vi "Graph Utilities Tree.vi"() -> ()   [LabVIEW 2019]
uses:
  graph_utilities.lvclass/graph_utilities.ctl
  <vilib>/Analysis/baseanly.llb/A x B.vi
  <vilib>/Analysis/baseanly.llb/A x Vector.vi
  subVIs/Step Average.vi
  <vilib>/Utility/error.llb/Error Cluster From Error Code.vi
  <vilib>/PRIrvin/XY Utilities/XY to 2D.vi
  graph_utilities.lvclass
panel:
  out "Intensity Graph":dbl[][](graph)
  out "XY Graph":cluster{dbl[], dbl[]}[](graph)
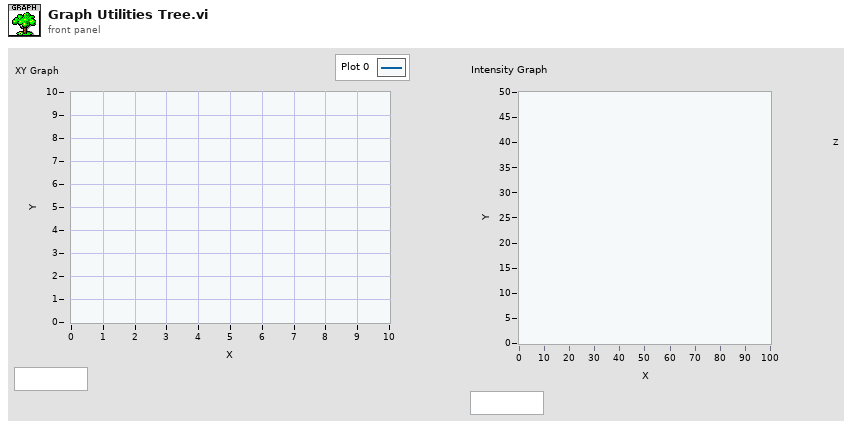
[diagram p1: front panel]
types:
  T1 = typedef "LVPointDoubleTypeDef.ctl" = cluster{"X":dbl, "Y":dbl}
  T2 = typedef "graph_utilities.lvclass/Scale Mapping --enum.ctl" = u16
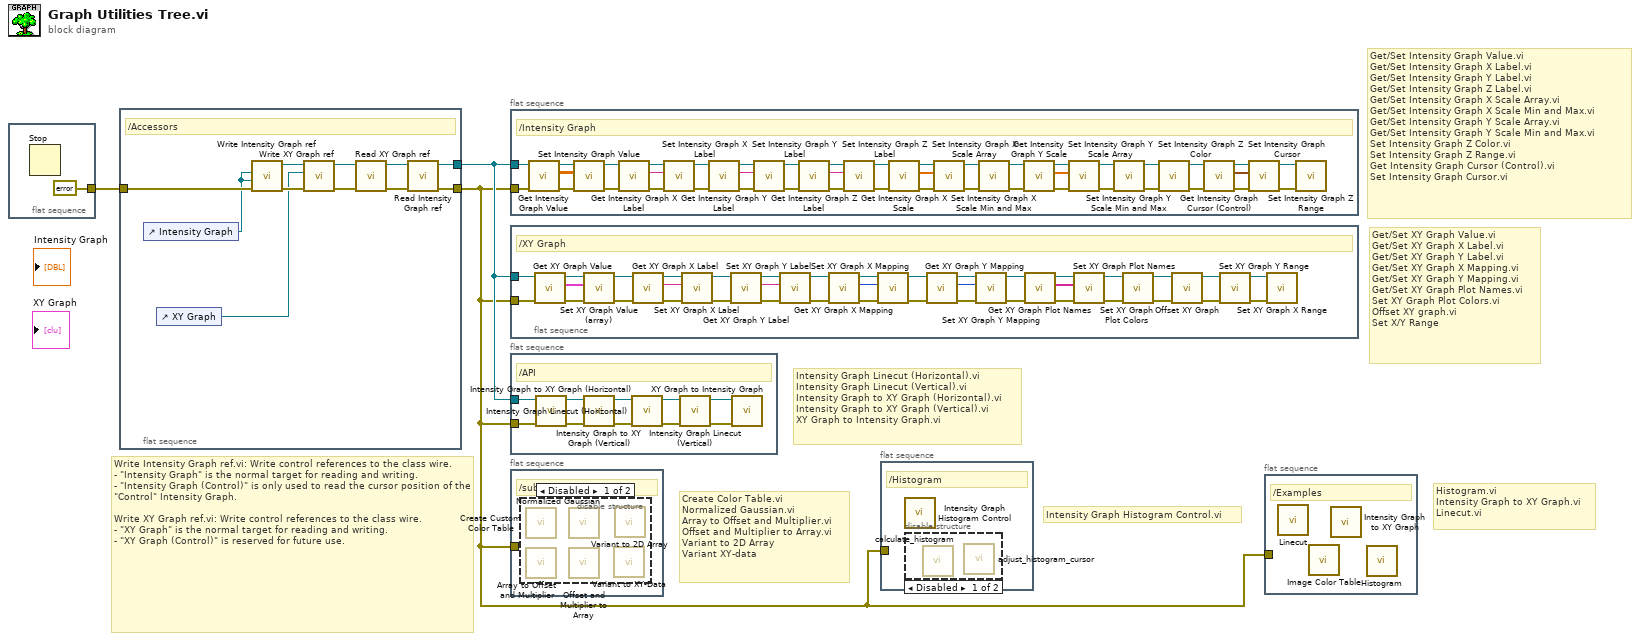
[diagram p0: block diagram]
diagram:
  # "Histogram.vi\nIntensity Graph to XY Graph.vi\nLinecut.vi"
  # "Intensity Graph Histogram Control.vi"
  # "Create Color Table.vi\nNormalized Gaussian.vi\nArray to Offset and Multiplier.vi\nOffset and Multiplier to Array.vi\nVariant to 2D Array\nVariant XY-data"
  # "Write Intensity Graph ref.vi: Write control references to the class wire.\n- \"Intensity Graph\" is the normal target for reading and writing.\n- \"Intensity Graph (Control)\" is only used to read the cursor position of the \"Control\" Intensity Graph.\n\nWrite XY Graph ref.vi: Write control references to the class wire.\n- \"XY Graph\" is the normal target for reading and writing.\n- \"XY Graph (Control)\" is reserved for future use."
  # "Get/Set Intensity Graph Value.vi\nGet/Set Intensity Graph X Label.vi\nGet/Set Intensity Graph Y Label.vi\nGet/Set Intensity Graph Z Label.vi\nGet/Set Intensity Graph X Scale Array.vi\nGet/Set Intensity Graph X Scale Min and Max.vi\nGet/Set Intensity Graph Y Scale Array.vi\nGet/Set Intensity Graph Y Scale Min and Max.vi\nSet Intensity Graph Z Color.vi\nSet Intensity Graph Z Range.vi\nGet Intensity Graph Cursor (Control).vi\nSet Intensity Graph Cursor.vi"
  # "Get/Set XY Graph Value.vi\nGet/Set XY Graph X Label.vi\nGet/Set XY Graph Y Label.vi\nGet/Set XY Graph X Mapping.vi\nGet/Set XY Graph Y Mapping.vi\nGet/Set XY Graph Plot Names.vi\nSet XY Graph Plot Colors.vi\nOffset XY graph.vi\nSet X/Y Range"
  # "Intensity Graph Linecut (Horizontal).vi\nIntensity Graph Linecut (Vertical).vi\nIntensity Graph to XY Graph (Horizontal).vi\nIntensity Graph to XY Graph (Vertical).vi\nXY Graph to Intensity Graph.vi"
  n1 = flat-sequence {
    tunnel: [errorcluster {"status"=FALSE, "code"=0, "source"=""} ("error in (no error)")] -> w3
    frame #0 {
      n2 = Stop() -> ()  [unwired: 1 in]
    }
  }
  n3 = flat-sequence {
    tunnel: w3 -> [w13]
    tunnel: [w8] -> w2
    tunnel: [w7] -> w1
    frame #0 {
      # "/Accessors"
      n4 = control-ref of="Intensity Graph"() -> (w6:refnum<vi>)
      n5 = control-ref of="XY Graph"() -> (w5:refnum<vi>)
      n6 = call "Write Intensity Graph ref.vi"("error in (no error)"=w13, "Intensity Graph (Control)"=w6, "Intensity Graph"=w6) -> ("error out"=w14:errorcluster, "graph_utilities out"=w15:refnum<class "graph_utilities.lvclass">)  [unwired: 7 in]
      n7 = call "Write XY Graph ref.vi"("error in (no error)"=w14, "XY Graph"=w5, "graph_utilities in"=w15) -> ("error out"=w12:errorcluster, "graph_utilities out"=w11:refnum<class "graph_utilities.lvclass">)  [unwired: 7 in]
      n8 = call "Read XY Graph ref.vi"("error in (no error)"=w12, "graph_utilities in"=w11) -> ("error out"=w9:errorcluster, "graph_utilities out"=w10:refnum<class "graph_utilities.lvclass">)  [unwired: 6 in, 2 out]
      n9 = call "Read Intensity Graph ref.vi"("error in (no error)"=w9, "graph_utilities in"=w10) -> ("error out"=w7:errorcluster, "graph_utilities out"=w8:refnum<class "graph_utilities.lvclass">)  [unwired: 6 in, 2 out]
    }
  }
  n10 = flat-sequence {
    tunnel: w2 -> [w27]
    tunnel: w1 -> [w26]
    frame #0 {
      # "/Intensity Graph"
      n11 = call "Get Intensity Graph Value.vi"("error in (no error)"=w26, "graph_utilities in"=w27) -> ("error out"=w56:errorcluster, "Value"=w58:dbl[][], "graph_utilities out"=w57:refnum<class "graph_utilities.lvclass">)  [unwired: 7 in]
      n12 = call "Set Intensity Graph Value.vi"("error in (no error)"=w56, "Value"=w58, "graph_utilities in"=w57) -> ("error out"=w54:errorcluster, "graph_utilities out"=w55:refnum<class "graph_utilities.lvclass">)  [unwired: 7 in]
      n13 = call "Get Intensity Graph X Label.vi"("error in (no error)"=w54, "graph_utilities in"=w55) -> ("error out"=w52:errorcluster, "X Label"=w37:string, "graph_utilities out"=w53:refnum<class "graph_utilities.lvclass">)  [unwired: 7 in]
      n14 = call "Set Intensity Graph X Label.vi"("error in (no error)"=w52, "X Label"=w37, "graph_utilities in"=w53) -> ("error out"=w50:errorcluster, "graph_utilities out"=w51:refnum<class "graph_utilities.lvclass">)  [unwired: 7 in]
      n15 = call "Get Intensity Graph Y Label.vi"("error in (no error)"=w50, "graph_utilities in"=w51) -> ("error out"=w48:errorcluster, "Y Label"=w36:string, "graph_utilities out"=w49:refnum<class "graph_utilities.lvclass">)  [unwired: 7 in]
      n16 = call "Set Intensity Graph Y Label.vi"("error in (no error)"=w48, "Y Label"=w36, "graph_utilities in"=w49) -> ("error out"=w46:errorcluster, "graph_utilities out"=w47:refnum<class "graph_utilities.lvclass">)  [unwired: 7 in]
      n17 = call "Get Intensity Graph Z Label.vi"("error in (no error)"=w46, "graph_utilities in"=w47) -> ("error out"=w44:errorcluster, "Z Label"=w35:string, "graph_utilities out"=w45:refnum<class "graph_utilities.lvclass">)  [unwired: 7 in]
      n18 = call "Set Intensity Graph Z Label.vi"("error in (no error)"=w44, "Z Label"=w35, "graph_utilities in"=w45) -> ("error out"=w42:errorcluster, "graph_utilities out"=w43:refnum<class "graph_utilities.lvclass">)  [unwired: 7 in]
      n19 = call "Get Intensity Graph X Scale.vi"("error in (no error)"=w42, "graph_utilities in"=w43) -> ("error out"=w40:errorcluster, "X Scale"=w34:dbl[], "graph_utilities out"=w41:refnum<class "graph_utilities.lvclass">)  [unwired: 6 in, 1 out]
      n20 = call "Set Intensity Graph X Scale Array.vi"("error in (no error)"=w40, "X Scale"=w34, "graph_utilities in"=w41) -> ("error out"=w24:errorcluster, "graph_utilities out"=w25:refnum<class "graph_utilities.lvclass">)  [unwired: 7 in]
      n21 = call "Set Intensity Graph X Scale Min and Max.vi"("error in (no error)"=w24, "graph_utilities in"=w25) -> ("error out"=w22:errorcluster, "graph_utilities out"=w23:refnum<class "graph_utilities.lvclass">)  [unwired: 8 in]
      n22 = call "Get Intensity Graph Y Scale.vi"("error in (no error)"=w22, "graph_utilities in"=w23) -> ("error out"=w38:errorcluster, "Y Scale"=w33:dbl[], "graph_utilities out"=w39:refnum<class "graph_utilities.lvclass">)  [unwired: 6 in, 1 out]
      n23 = call "Set Intensity Graph Y Scale Array.vi"("error in (no error)"=w38, "Y Scale"=w33, "graph_utilities in"=w39) -> ("error out"=w20:errorcluster, "graph_utilities out"=w21:refnum<class "graph_utilities.lvclass">)  [unwired: 7 in]
      n24 = call "Set Intensity Graph Y Scale Min and Max.vi"("error in (no error)"=w20, "graph_utilities in"=w21) -> ("error out"=w18:errorcluster, "graph_utilities out"=w19:refnum<class "graph_utilities.lvclass">)  [unwired: 8 in]
      n25 = call "Set Intensity Graph Z Color.vi"("error in (no error)"=w18, "graph_utilities in"=w19) -> ("error out"=w31:errorcluster, "graph_utilities out"=w30:refnum<class "graph_utilities.lvclass">)  [unwired: 8 in]
      n26 = call "Get Intensity Graph Cursor (Control).vi"("error in (no error)"=w31, "graph_utilities in"=w30) -> ("error out"=w29:errorcluster, "Cursor.Cursor Position"=w32:T1, "graph_utilities out"=w28:refnum<class "graph_utilities.lvclass">)  [unwired: 7 in]
      n27 = call "Set Intensity Graph Cursor.vi"("error in (no error)"=w29, "Cursor.Cursor Position"=w32, "graph_utilities in"=w28) -> ("error out"=w17:errorcluster, "graph_utilities out"=w16:refnum<class "graph_utilities.lvclass">)  [unwired: 7 in]
      n28 = call "Set Intensity Graph Z Range.vi"("error in (no error)"=w17, "graph_utilities in"=w16) -> ()  [unwired: 8 in, 2 out]
    }
  }
  n29 = flat-sequence {
    tunnel: w2 -> [w83]
    tunnel: w1 -> [w82]
    frame #0 {
      # "/XY Graph"
      n30 = call "Get XY Graph Value.vi"("error in (no error)"=w82, "graph_utilities in"=w83) -> ("error out"=w94:errorcluster, "XY-data"=w96:cluster{"X-array":dbl[], "Y-array":dbl[]}[], "graph_utilities out"=w95:refnum<class "graph_utilities.lvclass">)  [unwired: 7 in]
      n31 = call "Set XY Graph Value (array).vi"("error in (no error)"=w94, "XY-data"=w96, "graph_utilities in"=w95) -> ("error out"=w92:errorcluster, "graph_utilities out"=w93:refnum<class "graph_utilities.lvclass">)  [unwired: 7 in]
      n32 = call "Get XY Graph X Label.vi"("error in (no error)"=w92, "graph_utilities in"=w93) -> ("error out"=w90:errorcluster, "X Label"=w84:string, "graph_utilities out"=w91:refnum<class "graph_utilities.lvclass">)  [unwired: 7 in]
      n33 = call "Set XY Graph X Label.vi"("error in (no error)"=w90, "X Label"=w84, "graph_utilities in"=w91) -> ("error out"=w88:errorcluster, "graph_utilities out"=w89:refnum<class "graph_utilities.lvclass">)  [unwired: 7 in]
      n34 = call "Get XY Graph Y Label.vi"("error in (no error)"=w88, "graph_utilities in"=w89) -> ("error out"=w86:errorcluster, "Y Label"=w85:string, "graph_utilities out"=w87:refnum<class "graph_utilities.lvclass">)  [unwired: 7 in]
      n35 = call "Set XY Graph Y Label.vi"("error in (no error)"=w86, "Y Label"=w85, "graph_utilities in"=w87) -> ("error out"=w80:errorcluster, "graph_utilities out"=w81:refnum<class "graph_utilities.lvclass">)  [unwired: 7 in]
      n36 = call "Get XY Graph X Mapping.vi"("error in (no error)"=w80, "graph_utilities in"=w81) -> ("error out"=w78:errorcluster, "X Scale Mapping"=w65:T2, "graph_utilities out"=w79:refnum<class "graph_utilities.lvclass">)  [unwired: 7 in]
      n37 = call "Set XY Graph X Mapping.vi"("error in (no error)"=w78, "X Scale Mapping"=w65, "graph_utilities in"=w79) -> ("error out"=w76:errorcluster, "graph_utilities out"=w77:refnum<class "graph_utilities.lvclass">)  [unwired: 7 in]
      n38 = call "Get XY Graph Y Mapping.vi"("error in (no error)"=w76, "graph_utilities in"=w77) -> ("error out"=w74:errorcluster, "Y Scale Mapping"=w64:T2, "graph_utilities out"=w75:refnum<class "graph_utilities.lvclass">)  [unwired: 7 in]
      n39 = call "Set XY Graph Y Mapping.vi"("error in (no error)"=w74, "Y Scale Mapping"=w64, "graph_utilities in"=w75) -> ("error out"=w72:errorcluster, "graph_utilities out"=w73:refnum<class "graph_utilities.lvclass">)  [unwired: 7 in]
      n40 = call "Get XY Graph Plot Names.vi"("error in (no error)"=w72, "graph_utilities in"=w73) -> ("error out"=w70:errorcluster, "Plot Names []"=w63:string[], "graph_utilities out"=w71:refnum<class "graph_utilities.lvclass">)  [unwired: 7 in]
      n41 = call "Set XY Graph Plot Names.vi"("error in (no error)"=w70, "Plot Names []"=w63, "graph_utilities in"=w71) -> ("error out"=w68:errorcluster, "graph_utilities out"=w69:refnum<class "graph_utilities.lvclass">)  [unwired: 7 in]
      n42 = call "Set XY Graph Plot Colors.vi"("error in (no error)"=w68, "graph_utilities in"=w69) -> ("error out"=w66:errorcluster, "graph_utilities out"=w67:refnum<class "graph_utilities.lvclass">)  [unwired: 8 in]
      n43 = call "Offset XY Graph.vi"("error in (no error)"=w66, "graph_utilities in"=w67) -> ("error out"=w61:errorcluster, "graph_utilities out"=w62:refnum<class "graph_utilities.lvclass">)  [unwired: 8 in]
      n44 = call "Set XY Graph Y Range.vi"("error in (no error)"=w61, "graph_utilities in"=w62) -> ("error out"=w59:errorcluster, "graph_utilities out"=w60:refnum<class "graph_utilities.lvclass">)  [unwired: 8 in]
      n45 = call "Set XY Graph X Range.vi"("error in (no error)"=w59, "graph_utilities in"=w60) -> ()  [unwired: 8 in, 2 out]
    }
  }
  n46 = flat-sequence {
    tunnel: w2 -> [w98]
    tunnel: w1 -> [w97]
    frame #0 {
      # "/API"
      n47 = call "Intensity Graph to XY Graph (Horizontal).vi"("error in (no error)"=w97, "graph_utilities in"=w98) -> ("error out"=w105:errorcluster, "graph_utilities out"=w106:refnum<class "graph_utilities.lvclass">)  [unwired: 8 in]
      n48 = call "Intensity Graph to XY Graph (Vertical).vi"("error in (no error)"=w105, "graph_utilities in"=w106) -> ("error out"=w103:errorcluster, "graph_utilities out"=w104:refnum<class "graph_utilities.lvclass">)  [unwired: 8 in]
      n49 = call "Intensity Graph Linecut (Horizontal).vi"("error in (no error)"=w103, "graph_utilities in"=w104) -> ("error out"=w101:errorcluster, "graph_utilities out"=w102:refnum<class "graph_utilities.lvclass">)  [unwired: 8 in]
      n50 = call "Intensity Graph Linecut (Vertical).vi"("error in (no error)"=w101, "graph_utilities in"=w102) -> ("error out"=w99:errorcluster, "graph_utilities out"=w100:refnum<class "graph_utilities.lvclass">)  [unwired: 8 in]
      n51 = call "XY Graph to Intensity Graph.vi"("error in (no error)"=w99, "graph_utilities in"=w100) -> ()  [unwired: 8 in, 2 out]
    }
  }
  n52 = flat-sequence {
    tunnel: w1 -> [_]
    frame #0 {
      # "/subVIs"
      n53 = disable-structure shown="Disabled" {
        frame Disabled {
          n54 = call "Create Custom Color Table.vi"() -> ()  [unwired: 2 in, 4 out]
          n55 = call "Array to Offset and Multiplier.vi"() -> ()  [unwired: 1 in, 1 out]
          n56 = call "Normalized Gaussian.vi"() -> ()  [unwired: 10 in, 2 out]
          n57 = call "Offset and Multiplier to Array.vi"() -> ()  [unwired: 2 in, 1 out]
          n58 = call "Variant to XY-Data.vi"() -> ()  [unwired: 2 in, 2 out]
          n59 = call "Variant to 2D Array.vi"() -> ()  [unwired: 2 in, 2 out]
        }
        frame Enabled {
        }
      }
    }
  }
  n60 = flat-sequence {
    tunnel: w1 -> [_]
    frame #0 {
      # "/Histogram"
      n61 = call "Intensity Graph Histogram Control.vi"() -> ()  [unwired: 8 in, 4 out]
      n62 = disable-structure shown="Disabled" {
        frame Disabled {
          n63 = call "calculate_histogram.vi"() -> ()  [unwired: 8 in, 4 out]
          n64 = call "adjust_histogram_cursor.vi"() -> ()  [unwired: 10 in, 2 out]
        }
        frame Enabled {
        }
      }
    }
  }
  n65 = flat-sequence {
    tunnel: w1 -> [_]
    frame #0 {
      # "/Examples"
      n66 = call "Linecut.vi"() -> ()  [unwired: 12 in]
      n67 = call "Image Color Table.vi"() -> ()  [unwired: 12 in]
      n68 = call "Intensity Graph to XY Graph.vi"() -> ()  [unwired: 12 in]
      n69 = call "Histogram.vi"() -> ()  [unwired: 12 in]
    }
  }
